vi "sort mapping.vi"() -> ()   [LabVIEW 2018]
uses:
  <vilib>/Utility/file.llb/Read Delimited Spreadsheet (string).vi
panel:
  in  "Filter":string(combo)="Targets/Controller/Simulation Models/Models/Gear Model N/"
  out "system mapping filtered":string[][](array[string])=[["Aliases/altitude", "Targets/Controller/Simulation Models/Models/Gear Model N/Inports/Altitude"], ["Targets/Controller/Simulation Models/Models/ECU Model N/Outports/Torque DutyCycle", "Targets/Controller/Simulation Models/Models/Gear Model N/Inports/Torque"], ["Targets/Controller/Calculated Channels/Buzzer Check", "Targets/Controller/Simulation Models/Models/Gear Model N/Inports/Sleep"], ["Targets/Controller/Simulation Models/Models/Gear Model N/Outports/Gear Position", "Aliases/Test LGCU N Resolver"]]
  out "system mapping sorted":string[][](array[string])=[["Aliases/altitude", "Targets/Controller/Hardware/SLSC/SLSC Chassis/Modules/Slot 5 (SLSC SET Arinc429)/J1/ARINC Tx/CH 6/Altitude/Word/Altitude"], ["Targets/Controller/Simulation Models/Models/ECU Model N/Outports/Torque DutyCycle", "Targets/Controller/Custom Devices/FPGA Addon/Scalars/Scalar Outputs/Nose Torque (0-1)"], ["Targets/Controller/Calculated Channels/Panel RealSim Up Command", "Targets/Controller/Custom Devices/Switch/Discretes/Test LGCU Panel UP Command"], ["Targets/Controller/Calculated Channels/Panel RealSim Down Command", "Targets/Controller/Custom Devices/Switch/Discretes/Test LGCU Panel Down Command"], ["Targets/Controller/User Channels/Power", "Targets/Controller/Custom Devices/Switch/Discretes/Test LGCU Ground "], ["Targets/Controller/Calculated Channels/Gear Fault Open//Connected", "Targets/Controller/Custom Devices/Switch/InputStates/Test LGCU N Motor Current State1"], ["Targets/Controller/Calculated Channels/Groupswitch Gear", "Targets/Controller/Custom Devices/Group Switching/Gear RealSim/Gear RealSim Switch"], ["Targets/Controller/Calculated Channels/Groupswitch Panel", "Targets/Controller/Custom Devices/Group Switching/Panel RealSim/Panel RealSim Switch"], ["Targets/Controller/User Channels/Power", "Targets/Controller/Custom Devices/Group Switching/SimStates/SimStates Switch"], ["Aliases/altitude", "Targets/Controller/Custom Devices/LGCU Interrogation Port/Altitude_000"], ["Aliases/altitude", "Targets/Controller/Simulation Models/Models/Gear Model N/Inports/Altitude"], ["Targets/Controller/Simulation Models/Models/ECU Model N/Outports/Torque DutyCycle", "Targets/Controller/Simulation Models/Models/Gear Model N/Inports/Torque"], ["Targets/Controller/Calculated Channels/Buzzer Check", "Targets/Controller/Simulation Models/Models/Gear Model N/Inports/Sleep"], ["Aliases/altitude", "Targets/Controller/Simulation Models/Models/Gear Model LR/Inports/Altitude"], ["Aliases/Proto LGCU Panel Down Command", "Targets/Controller/Simulation Models/Models/ECU Model N/Inports/ Gear Up Command"], ["Aliases/Proto LGCU Panel UP Command", "Targets/Controller/Simulation Models/Models/ECU Model N/Inports/ Gear Down Command"], ["Targets/Controller/User Channels/Sleep", "Targets/Controller/Simulation Models/Models/ECU Model N/Inports/Sleep In"], ["Aliases/Proto LGCU N Resolver", "Targets/Controller/Simulation Models/Models/ECU Model N/Inports/ Gear Position"], ["Aliases/altitude", "Targets/Controller/Simulation Models/Models/ECU Model N/Inports/Altitude"], ["Targets/Controller/Simulation Models/Models/Gear Model N/Outports/Gear Position", "Aliases/Test LGCU N Resolver"], ["Targets/Controller/User Channels/Power", "Aliases/Proto LGCU 28V Power A"], ["Targets/Controller/Simulation Models/Models/ECU Model N/Outports/Panel Lamp G", "Aliases/Proto LGCU L Lamp G"], ["Targets/Controller/Simulation Models/Models/ECU Model N/Outports/Panel Lamp R", "Aliases/Proto LGCU L Lamp R"], ["Targets/Controller/Simulation Models/Models/ECU Model N/Outports/Panel Lamp G", "Aliases/Proto LGCU N Lamp G"], ["Targets/Controller/Simulation Models/Models/ECU Model N/Outports/Panel Lamp R", "Aliases/Proto LGCU N Lamp R"], ["Targets/Controller/User Channels/Power", "Aliases/Proto LGCU IND GRN"], ["Targets/Controller/Calculated Channels/Error", "Aliases/Proto LGCU Error Lamp"], ["Targets/Controller/Calculated Channels/Buzzer Check", "Aliases/Proto LGCU Buzz"], ["Targets/Controller/User Channels/Power", "Aliases/Proto DCU IND GRN"], ["Targets/Controller/User Channels/altitude", "Aliases/altitude"]]
  out "system mapping":string[][](array[string])=[["Aliases/altitude", "Targets/Controller/Hardware/SLSC/SLSC Chassis/Modules/Slot 5 (SLSC SET Arinc429)/J1/ARINC Tx/CH 6/Altitude/Word/Altitude"], ["Targets/Controller/Simulation Models/Models/ECU Model N/Outports/Torque DutyCycle", "Targets/Controller/Custom Devices/FPGA Addon/Scalars/Scalar Outputs/Nose Torque (0-1)"], ["Targets/Controller/Calculated Channels/Panel RealSim Up Command", "Targets/Controller/Custom Devices/Switch/Discretes/Test LGCU Panel UP Command"], ["Targets/Controller/Calculated Channels/Panel RealSim Down Command", "Targets/Controller/Custom Devices/Switch/Discretes/Test LGCU Panel Down Command"], ["Targets/Controller/User Channels/Power", "Targets/Controller/Custom Devices/Switch/Discretes/Test LGCU Ground "], ["Targets/Controller/Calculated Channels/Gear Fault Open//Connected", "Targets/Controller/Custom Devices/Switch/InputStates/Test LGCU N Motor Current State1"], ["Targets/Controller/Calculated Channels/Groupswitch Gear", "Targets/Controller/Custom Devices/Group Switching/Gear RealSim/Gear RealSim Switch"], ["Targets/Controller/Calculated Channels/Groupswitch Panel", "Targets/Controller/Custom Devices/Group Switching/Panel RealSim/Panel RealSim Switch"], ["Targets/Controller/User Channels/Power", "Targets/Controller/Custom Devices/Group Switching/SimStates/SimStates Switch"], ["Aliases/altitude", "Targets/Controller/Custom Devices/LGCU Interrogation Port/Altitude_000"], ["Aliases/altitude", "Targets/Controller/Simulation Models/Models/Gear Model N/Inports/Altitude"], ["Targets/Controller/Simulation Models/Models/ECU Model N/Outports/Torque DutyCycle", "Targets/Controller/Simulation Models/Models/Gear Model N/Inports/Torque"], ["Targets/Controller/Calculated Channels/Buzzer Check", "Targets/Controller/Simulation Models/Models/Gear Model N/Inports/Sleep"], ["Aliases/altitude", "Targets/Controller/Simulation Models/Models/Gear Model LR/Inports/Altitude"], ["Aliases/Proto LGCU Panel Down Command", "Targets/Controller/Simulation Models/Models/ECU Model N/Inports/ Gear Up Command"], ["Aliases/Proto LGCU Panel UP Command", "Targets/Controller/Simulation Models/Models/ECU Model N/Inports/ Gear Down Command"], ["Targets/Controller/User Channels/Sleep", "Targets/Controller/Simulation Models/Models/ECU Model N/Inports/Sleep In"], ["Aliases/Proto LGCU N Resolver", "Targets/Controller/Simulation Models/Models/ECU Model N/Inports/ Gear Position"], ["Aliases/altitude", "Targets/Controller/Simulation Models/Models/ECU Model N/Inports/Altitude"], ["Targets/Controller/Simulation Models/Models/Gear Model N/Outports/Gear Position", "Aliases/Test LGCU N Resolver"], ["Targets/Controller/User Channels/Power", "Aliases/Proto LGCU 28V Power A"], ["Targets/Controller/Simulation Models/Models/ECU Model N/Outports/Panel Lamp G", "Aliases/Proto LGCU L Lamp G"], ["Targets/Controller/Simulation Models/Models/ECU Model N/Outports/Panel Lamp R", "Aliases/Proto LGCU L Lamp R"], ["Targets/Controller/Simulation Models/Models/ECU Model N/Outports/Panel Lamp G", "Aliases/Proto LGCU N Lamp G"], ["Targets/Controller/Simulation Models/Models/ECU Model N/Outports/Panel Lamp R", "Aliases/Proto LGCU N Lamp R"], ["Targets/Controller/User Channels/Power", "Aliases/Proto LGCU IND GRN"], ["Targets/Controller/Calculated Channels/Error", "Aliases/Proto LGCU Error Lamp"], ["Targets/Controller/Calculated Channels/Buzzer Check", "Aliases/Proto LGCU Buzz"], ["Targets/Controller/User Channels/Power", "Aliases/Proto DCU IND GRN"], ["Targets/Controller/User Channels/altitude", "Aliases/altitude"]]
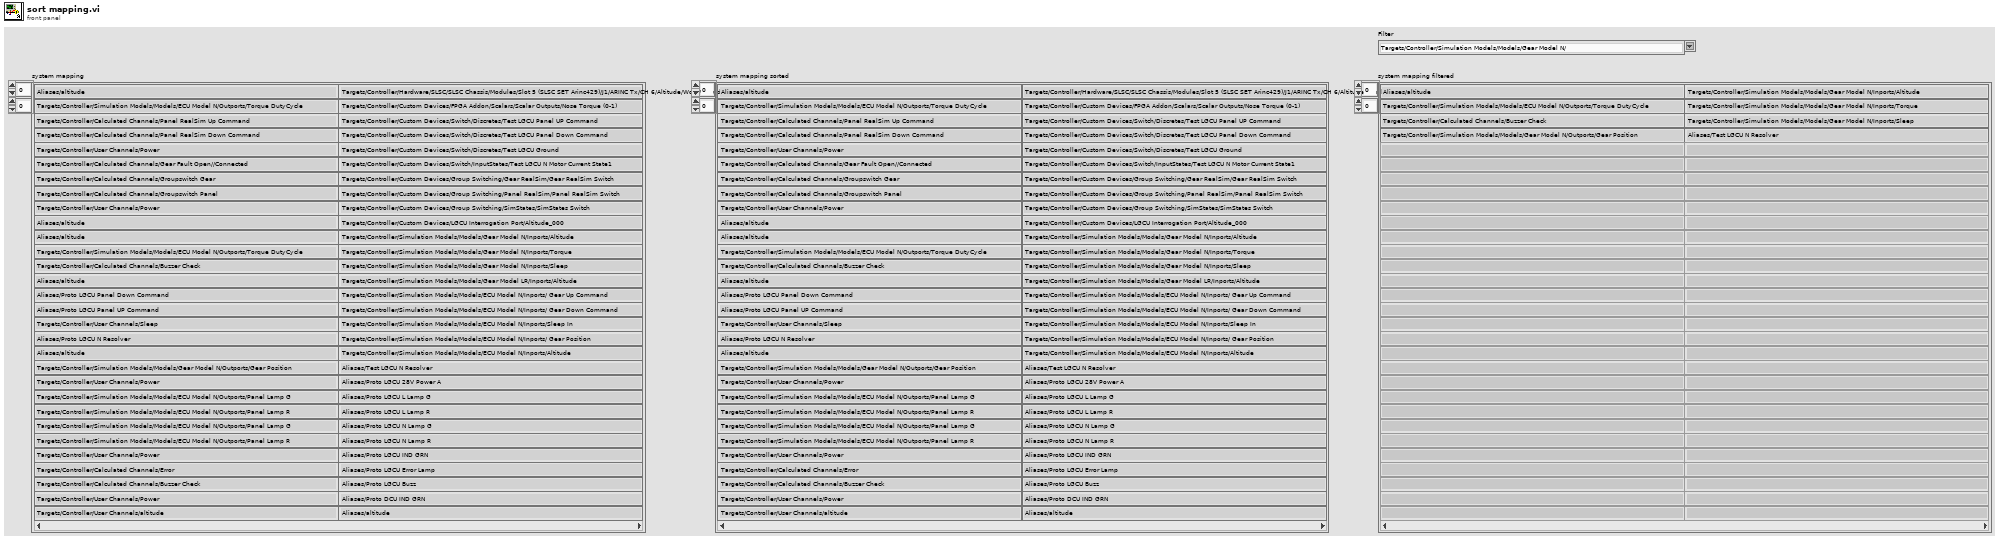
[diagram p1: front panel]
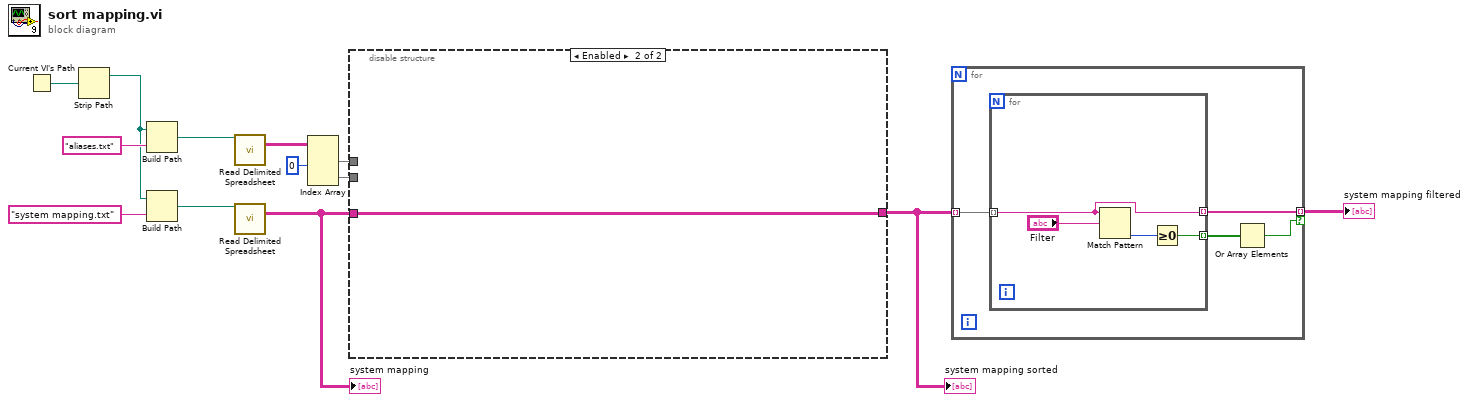
[diagram p0: block diagram]
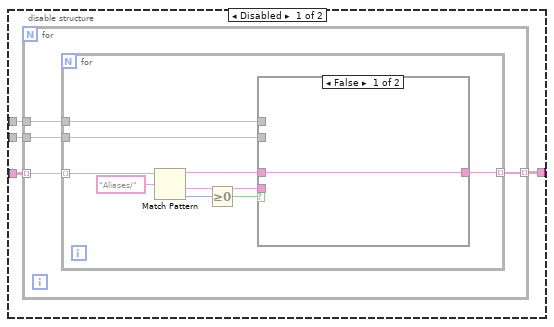
[diagram p2: hidden frame]
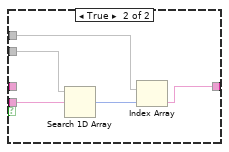
[diagram p3: hidden frame]
diagram:
  n1 = Current VI's Path() -> (path=w13:path)
  n2 = Strip Path(path=w13) -> (stripped path=w10:path)  [unwired: 1 out]
  n3 = Build Path(base path=w10, name or relative path="aliases.txt") -> (appended path=w8:path)
  n4 = Build Path(base path=w10, name or relative path="system mapping.txt") -> (appended path=w9:path)
  n5 = call-poly <vilib>:"Read Delimited Spreadsheet.vi"("file path (dialog if empty)"=w8) -> ("all rows"=w7:string[][])  [unwired: 9 in, 5 out]
  n6 = call-poly <vilib>:"Read Delimited Spreadsheet.vi"("file path (dialog if empty)"=w9) -> ("all rows"=w3:string[][])  [unwired: 9 in, 5 out]
  "system mapping" <- w3
  n7 = Index Array(array=w7, index (col) #1=0 ("disabled index (col)")) -> (element #1=w5:string[], element #2=w4:string[])  [unwired: 3 in]
  n8 = disable-structure shown="Enabled" {
    disable-tunnel: w5 -> [w17 _]
    disable-tunnel: w4 -> [w16 _]
    disable-tunnel: w3 -> [w15 w37]
    disable-tunnel: [w14 w37] -> w2
    frame Disabled {
      n9 = for {
        tunnel: w17 -> [w21]
        tunnel: w16 -> [w20]
        tunnel: [w19] -> w14 mode=indexing
        tunnel: w15 -> [w18] mode=indexing
        n10 = for {
          tunnel: w18 -> [w30] mode=indexing
          tunnel: w21 -> [w26]
          tunnel: w20 -> [w25]
          tunnel: [w23] -> w19 mode=indexing
          n11 = Match Pattern(string=w30, regular expression="Aliases/") -> (before substring=w24:string, after substring=w22:string, offset past match=w28:i32)  [unwired: 1 in, 1 out]
          n12 = Greater Or Equal To 0?(x=w28) -> (x >= 0?=w27:bool)
          n13 = case shown="False" w27 {
            tunnel: w26 -> [_ w32]
            tunnel: w25 -> [_ w33]
            tunnel: w24 -> [w31 _]
            tunnel: [w31 w34] -> w23
            tunnel: w22 -> [_ w36]
            frame False {
            }
            frame True {
              n14 = Search 1D Array(1D array=w33, element=w36) -> (index of element=w35:i32)  [unwired: 1 in]
              n15 = Index Array(array=w32, index=w35) -> (element=w34:string)
            }
          }
        }
      }
    }
    frame Enabled {
    }
  }
  "system mapping sorted" <- w2
  n16 = for {
    tunnel: [w41] -> w1 mode=indexing if=w38
    tunnel: w2 -> [w40] mode=indexing
    n17 = for {
      tunnel: w40 -> [w43] mode=indexing
      tunnel: [w43] -> w41 mode=indexing
      tunnel: [w44] -> w39 mode=indexing
      n18 = Match Pattern(string=w43, regular expression="Filter") -> (offset past match=w45:i32)  [unwired: 1 in, 3 out]
      n19 = Greater Or Equal To 0?(x=w45) -> (x >= 0?=w44:bool)
    }
    n20 = Or Array Elements(Boolean array=w39) -> (logical OR=w38:bool)
  }
  "system mapping filtered" <- w1
